vi "Voltage pulses at various Z.vi"() -> ()   [LabVIEW 2016]
doc: "This example applies bias voltage pulses at various Z positions.\n\n- Nanonis Programming Interface -"
uses:
  Nanonis Prog Interface.lvlib
panel:
  in  "Pulse width (s)":dbl=0.1 min=0.0 max=100.0 format="%#_6p"
  in  "Bias pulse (V)":dbl=5.0 min=-10.0 max=10.0
  in  "Z steps number":u16=10 min=1
  in  "Delta Z (m)":dbl=9.999999717180685e-10 format="%#_6p"
  out "Current Z":dbl caption="Current Z position (m)" format="%#_5p"
  # "Example program for the Nanonis SPM Control software programming interface\n\n- Apply bias voltage pulses at various Z -"
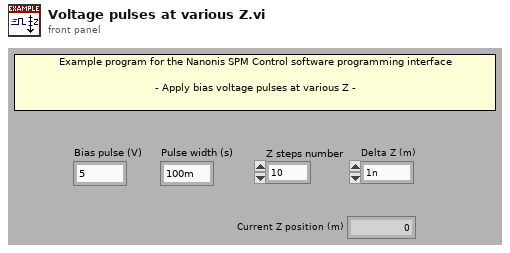
[diagram p1: front panel]
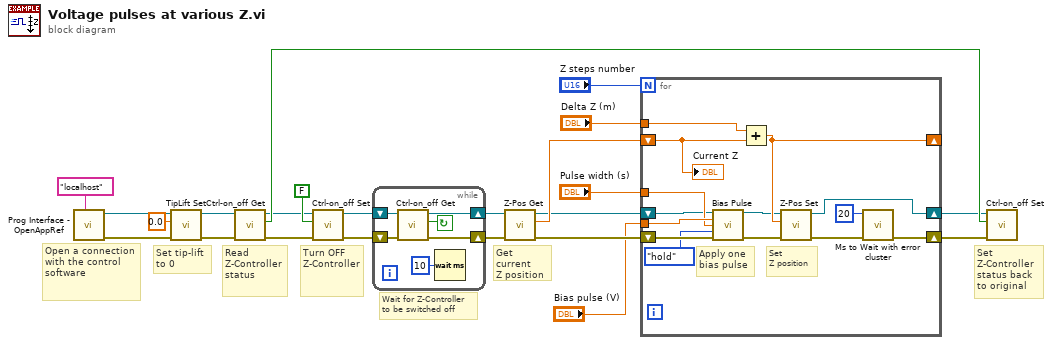
[diagram p0: block diagram]
diagram:
  # "Wait for Z-Controller\nto be switched off"
  # "Set \nZ-Controller\nstatus back to original"
  # "Get current\nZ position"
  # "Turn OFF \nZ-Controller"
  # "Read \nZ-Controller\nstatus"
  # "Set tip-lift\nto 0"
  # "Open a connection with the control\nsoftware"
  n1 = call <userlib>:"Prog Interface - OpenAppRef.vi"("Machine name (local machine IP)"="localhost" ("machine name (localhost)")) -> ("Error out"=w23:errorcluster, "Application reference"=w7:refnum<vi>)  [unwired: 5 in]
  n2 = call <userlib>:"TipLift Set.vi"("error in (no error)"=w23, "TipLift (m)"=sgl 0.0, "Application ref in"=w7) -> ("error out"=w20:errorcluster, "Application ref out"=w6:refnum<vi>)  [unwired: 7 in]
  n3 = call <userlib>:"Ctrl-on_off Get.vi"("error in (no error)"=w20, "Application ref in"=w6) -> ("error out"=w18:errorcluster, "Z-Controller on/off status"=w13:bool, "Application ref out"=w5:refnum<vi>)  [unwired: 7 in]
  n4 = call <userlib>:"Ctrl-on_off Set.vi"("error in (no error)"=w18, "Z Controller ON/OFF"=FALSE ("Ctrl on/off"), "Application ref in"=w5) -> ("error out"=w9:errorcluster, "Application ref out"=w4:refnum<vi>)  [unwired: 7 in]
  n5 = while {
    shift-right: [w29] -> w8
    shift-left: w9 -> [w28]
    shift-right: [w24] -> w3
    shift-left: w4 -> [w25]
    stop <- w27 continue-if-true
    n6 = call <userlib>:"Ctrl-on_off Get.vi"("error in (no error)"=w28, "Application ref in"=w25) -> ("error out"=w29:errorcluster, "Z-Controller on/off status"=w27:bool, "Application ref out"=w24:refnum<vi>)  [unwired: 7 in]
    n7 = Wait (ms)(milliseconds to wait=u32 10) -> ()  [unwired: 1 out]
  }
  n8 = call <userlib>:"Z-Pos Get.vi"("error in (no error)"=w8, "Application ref in"=w3) -> ("error out"=w16:errorcluster, "Z position (m)"=w15:sgl, "Application ref out"=w2:refnum<vi>)  [unwired: 7 in]
  n9 = for {
    N: "Z steps number" -> [_]
    shift-right: [w41] -> _
    shift-left: w15 -> [w40]
    shift-right: [w33] -> w14
    shift-left: w16 -> [w43]
    tunnel: "Bias pulse (V)" -> [w38]
    tunnel: "Pulse width (s)" -> [w37]
    tunnel: "Delta Z (m)" -> [w36]
    shift-right: [w30] -> w1
    shift-left: w2 -> [w32]
    # "Set\nZ position"
    # "Apply one bias pulse"
    n10 = call <userlib>:"Bias Pulse.vi"("Application ref in"=w32, "Pulse bias (V) (1)"=w38, "Pulse width (s) (100m)"=w37, "Z-Controller (no change)"=enum16{"no change", "hold", "don't hold"}."hold", "Error in (no error)"=w43) -> ("Application ref out"=w31:refnum<vi>, "Error out"=w42:errorcluster)  [unwired: 9 in]
    n11 = Add(x=w36, y=w40) -> (x+y=w41:dbl)
    n12 = call <userlib>:"Z-Pos Set.vi"("error in (no error)"=w42, "Z position (m)"=w41, "Application ref in"=w31) -> ("error out"=w34:errorcluster, "Application ref out"=w30:refnum<vi>)  [unwired: 7 in]
    n13 = call "Ms to Wait with error cluster.vi"("error in (no error)"=w34, "milliseconds to wait"=u32 20) -> ("error out"=w33:errorcluster)  [unwired: 4 in, 1 out]
    "Current Z" <- w40
  }
  n14 = call <userlib>:"Ctrl-on_off Set.vi"("error in (no error)"=w14, "Z Controller ON/OFF"=w13, "Application ref in"=w1) -> ()  [unwired: 7 in, 2 out]
